vi "KNRmOS6Delta Linear movement.vi"(8 "error in (no error)":errorcluster, 9 "z0":dbl(slide) scale=-135.0..50.0, 10 "y0":dbl(slide) scale=-115.0..115.0, 11 "x0":dbl(slide) scale=-115.0..115.0) -> (0 "error out":errorcluster)   [LabVIEW 2019]
uses:
  math/Global 1.vi
panel:
  out "non-existing point":bool
  out "thetaY":dbl
  out "thetaX":dbl
  out "thetaZ":dbl
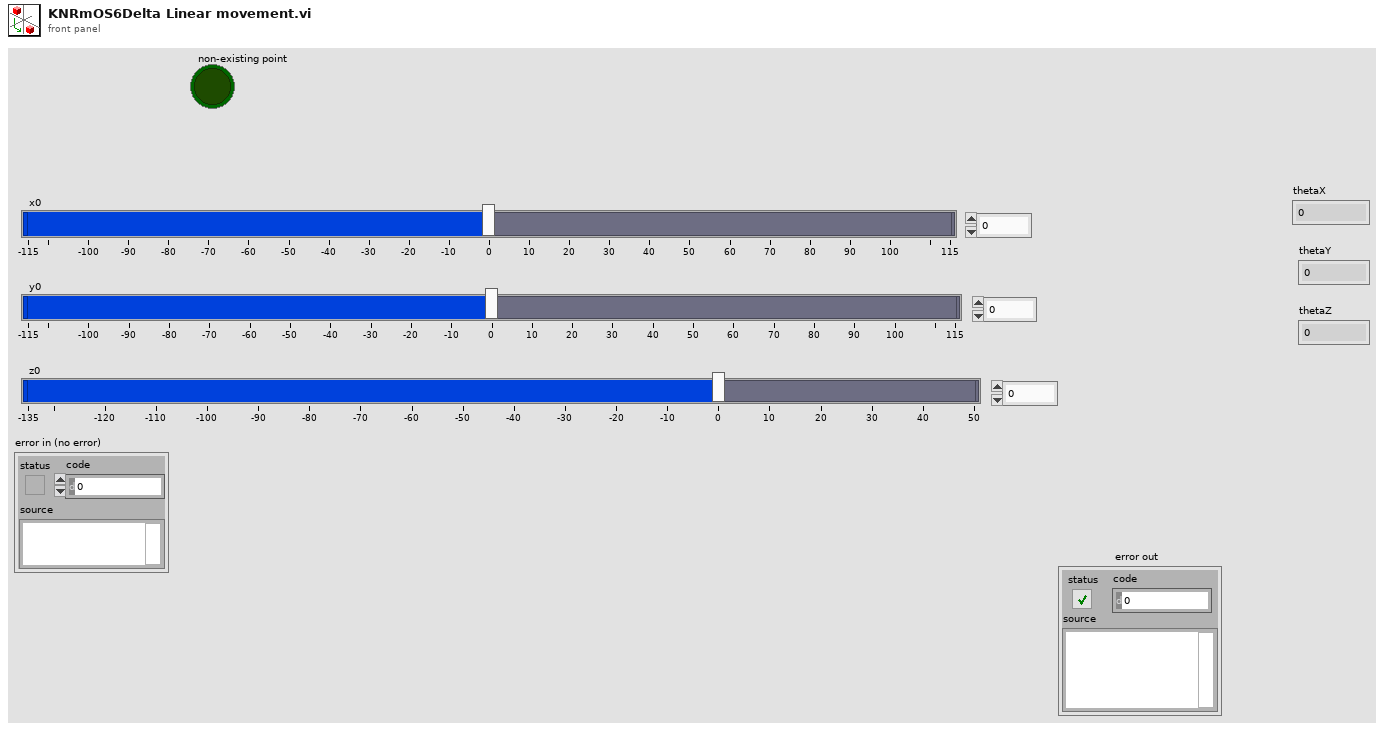
[diagram p1: front panel]
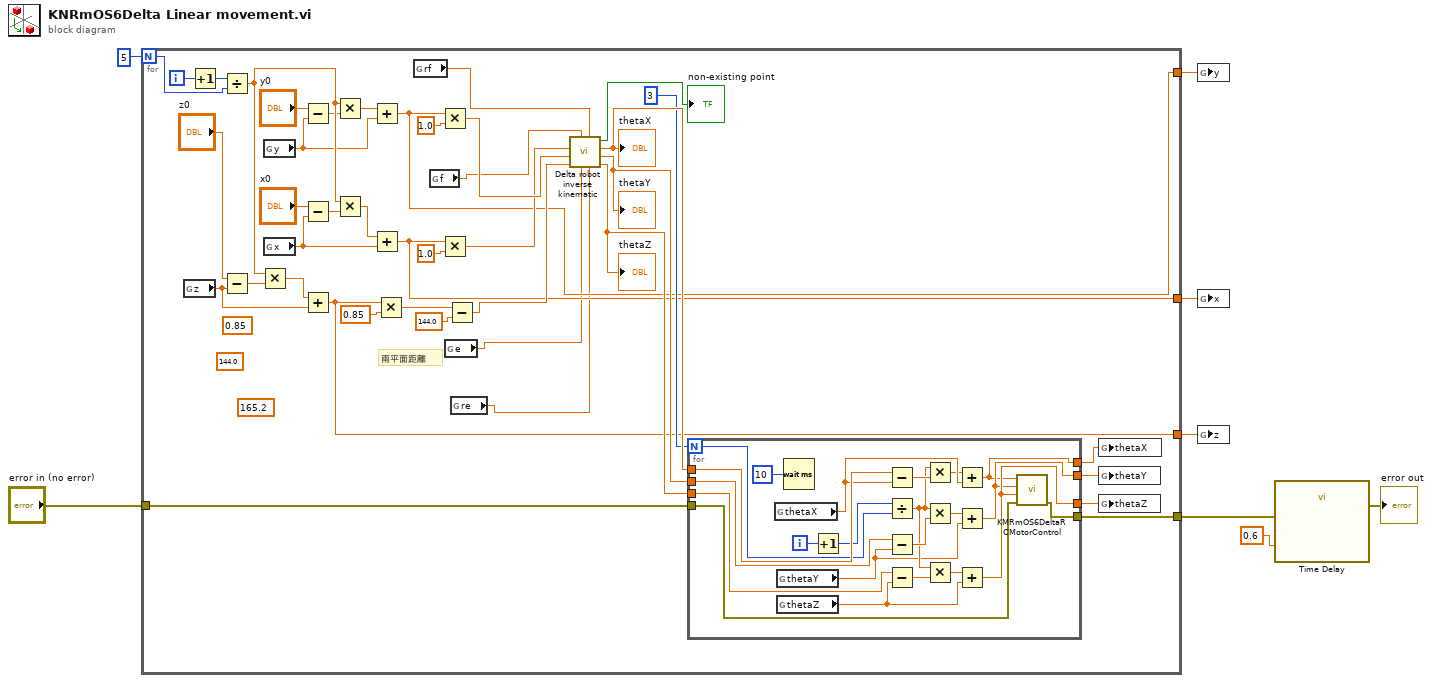
[diagram p0: block diagram]
diagram:
  n1 = for {
    N: 5 -> [w17]
    tunnel: [w33] -> w4
    tunnel: [w16] -> w7
    tunnel: [w15] -> w6
    tunnel: [w14] -> w5
    tunnel: "error in (no error)" -> [w13]
    i -> [w18]
    (unwired) 165.2 ("y")
    (unwired) 0.85 ("y")
    (unwired) 144.0 ("y")
    # "兩平面距離"
    n2 = global read "Global 1.vi" "z"() -> (w23:dbl)
    n3 = Increment(x=w18) -> (x+1=w25:i32)
    n4 = Divide(x=w25, y=w17) -> (x/y=w31:dbl)
    n5 = Subtract(x="z0", y=w23) -> (x-y=w32:dbl)
    n6 = Multiply(x=w31, y=w32) -> (x*y=w29:dbl)
    n7 = global read "Global 1.vi" "y"() -> (w21:dbl)
    n8 = global read "Global 1.vi" "x"() -> (w20:dbl)
    n9 = Subtract(x="y0", y=w21) -> (x-y=w30:dbl)
    n10 = Subtract(x="x0", y=w20) -> (x-y=w26:dbl)
    n11 = Add(x=w29, y=w23) -> (x+y=w14:dbl)
    n12 = Multiply(x=w31, y=w30) -> (x*y=w28:dbl)
    n13 = Multiply(x=w31, y=w26) -> (x*y=w27:dbl)
    n14 = Add(x=w28, y=w21) -> (x+y=w15:dbl)
    n15 = Add(x=w27, y=w20) -> (x+y=w16:dbl)
    n16 = Multiply(x=w14, y=0.85) -> (x*y=w36:dbl)
    n17 = global read "Global 1.vi" "rf"() -> (w12:dbl)
    n18 = global read "Global 1.vi" "f"() -> (w11:dbl)
    n19 = Multiply(x=w15, y=1.0) -> (x*y=w41:dbl)
    n20 = Multiply(x=w16, y=1.0) -> (x*y=w39:dbl)
    n21 = global read "Global 1.vi" "e"() -> (w10:dbl)
    n22 = Subtract(x=w36, y=144.0) -> (x-y=w34:dbl)
    n23 = global read "Global 1.vi" "re"() -> (w9:dbl)
    n24 = call "Delta robot inverse kinematic.vi"("re"=w9, "rf"=w12, "e"=w10, "f"=w11, "z0"=w34, "y0"=w41, "x0"=w39) -> ("thetaZ"=w47:dbl, "thetaY"=w48:dbl, "thetaX"=w49:dbl, "non-existing point"=→"non-existing point":bool)  [unwired: 1 in]
    "thetaZ" <- w47
    "thetaX" <- w49
    "thetaY" <- w48
    n25 = for {
      N: 3 -> [w64]
      tunnel: w49 -> [w70]
      tunnel: w48 -> [w69]
      tunnel: w47 -> [w68]
      tunnel: [w52] -> w45
      tunnel: [w54] -> w44
      tunnel: [w53] -> w43
      tunnel: w13 -> [w51]
      tunnel: [w50] -> w33
      i -> [w66]
      n26 = global read "Global 1.vi" "thetaX"() -> (w67:dbl)
      n27 = global read "Global 1.vi" "thetaY"() -> (w56:dbl)
      n28 = global read "Global 1.vi" "thetaZ"() -> (w55:dbl)
      n29 = Wait (ms)(milliseconds to wait=u32 10) -> ()  [unwired: 1 out]
      n30 = Increment(x=w66) -> (x+1=w65:i32)
      n31 = Subtract(x=w70, y=w67) -> (x-y=w63:dbl)
      n32 = Divide(x=w65, y=w64) -> (x/y=w58:dbl)
      n33 = Subtract(x=w69, y=w56) -> (x-y=w59:dbl)
      n34 = Subtract(x=w68, y=w55) -> (x-y=w57:dbl)
      n35 = Multiply(x=w58, y=w63) -> (x*y=w62:dbl)
      n36 = Multiply(x=w58, y=w59) -> (x*y=w61:dbl)
      n37 = Multiply(x=w58, y=w57) -> (x*y=w60:dbl)
      n38 = Add(x=w62, y=w67) -> (x+y=w52:dbl)
      n39 = Add(x=w61, y=w56) -> (x+y=w53:dbl)
      n40 = Add(x=w60, y=w55) -> (x+y=w54:dbl)
      n41 = call "KMRmOS6DeltaRCMotorControl.vi"("error in (no error)"=w51, "Theta3"=w54, "Theta2"=w53, "Theta1"=w52) -> ("error out"=w50:errorcluster)  [unwired: 7 in]
    }
    n42 = global write "Global 1.vi" "thetaX"(w45) -> ()
    n43 = global write "Global 1.vi" "thetaY"(w43) -> ()
    n44 = global write "Global 1.vi" "thetaZ"(w44) -> ()
  }
  n45 = global write "Global 1.vi" "y"(w6) -> ()
  n46 = global write "Global 1.vi" "x"(w7) -> ()
  n47 = global write "Global 1.vi" "z"(w5) -> ()
  n48 = call "Time Delay"("error in (no error)"=w4, "Delay Time (s)"=0.6) -> ("error out"=→"error out":errorcluster)  [unwired: 9 in]
